vi "Design a Fixed-Point Interpolation Multirate Filter.vi"() -> ()   [LabVIEW 2023]
uses:
  <vilib>/addons/Digital Filter Design/FXPMRateSim.llb/DFD FXP MRate Simulation (DBL).vi
  <vilib>/addons/Digital Filter Design/FilterLib.llb/DFD Save MRate Filter to File.vi
  <vilib>/addons/Digital Filter Design/NI_DigFilterLicensed.lvlib
panel:
  out "Error Message":string
  in  "Save Filter to File":bool
  in  "Signal from DAQ Device":fxp<+/-,20,5>[](array[numeric])=[-0.329681396484375, -4.286834716796875, 9.429473876953125, -8.305145263671875, -0.662689208984375, -2.729522705078125, 7.085845947265625, -3.488800048828125, 2.225128173828125, 3.63323974609375, -5.179962158203125, 7.238677978515625, 4.8243408203125, 2.791412353515625, -9.072296142578125, -1.45458984375, 9.80548095703125, 7.69830322265625, -9.72210693359375, 1.994598388671875, -6.56597900390625, 5.69097900390625, 8.246246337890625, -2.866546630859375, -6.74896240234375, -7.206298828125, -4.030517578125, 6.043731689453125, 8.05010986328125, 3.516815185546875, 9.917205810546875, -8.699188232421875, 0.4688720703125, 0.513763427734375, 4.93695068359375, 5.129974365234375, -7.52783203125, 7.8001708984375, 1.576171875, 2.575714111328125, -4.20550537109375, -1.79620361328125, -5.672332763671875, 7.192901611328125, 9.375030517578125, -2.6258544921875, -5.70220947265625, 4.27691650390625, -0.683868408203125, 4.7548828125, 7.179962158203125, 7.098846435546875, -4.2564697265625, -8.908050537109375, -3.31884765625, 5.65350341796875, 0.428924560546875, 1.617706298828125, 7.4306640625, 4.920562744140625, -7.7008056640625, -7.17559814453125, -4.438934326171875, 8.03948974609375, 6.6856689453125, -2.220062255859375, -5.266357421875, -9.69549560546875, -7.25823974609375, 3.82177734375, 6.288909912109375, -1.042572021484375, 1.600128173828125, 8.114593505859375, 3.807037353515625, 7.95660400390625, -4.94366455078125, 0.53521728515625, 5.354522705078125, 5.111419677734375, 5.87420654296875, 5.844146728515625, 7.76446533203125, 6.58843994140625, 2.994964599609375, 0.97381591796875, 4.075286865234375, -2.38446044921875, -8.872802734375, 7.240264892578125, 3.440216064453125, -3.22064208984375, 7.457244873046875, -8.672027587890625, -7.299957275390625, -7.650421142578125, -8.7384033203125, -2.68670654296875, -0.992645263671875, 7.793701171875, -7.697601318359375, -1.930633544921875, 7.630767822265625, 8.330291748046875, -8.08685302734375, -8.128021240234375, 2.206024169921875, -2.2911376953125, -7.6170654296875, -6.148284912109375, -9.52166748046875, -5.676300048828125, 9.081939697265625, -1.682403564453125, -0.28973388671875, 2.24139404296875, -2.659698486328125, -9.855255126953125, 1.220489501953125, 2.930938720703125, 9.869171142578125, -2.096160888671875, 4.275848388671875, 0.7493896484375, 7.155364990234375, 8.169921875, 2.828765869140625, 8.2470703125] format="%.6g"
  out "Filtered Signals":dbl[](graph)
  # "Design a fixed-point highpass interpolation filter"
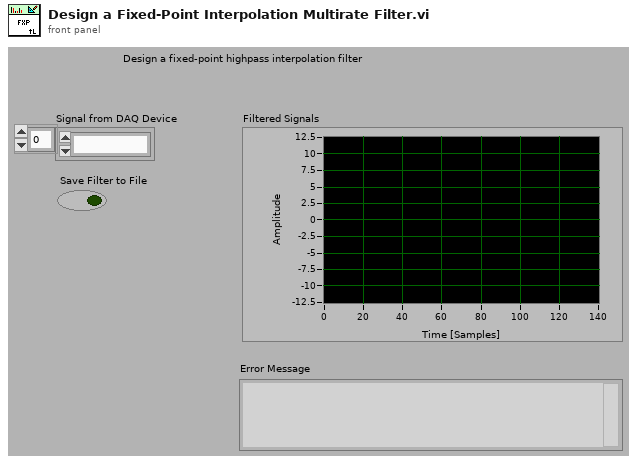
[diagram p1: front panel]
types:
  T1 = typedef "NI_DigFilterLicensed.lvlib/DFD Multirate Filter Obj.ctl" = cluster{"mMRate_Structure":enum16{"CIC", "FIR", "IIR", "Lattice"}, "mMRate_Mode":T2, "mMRate_Factor":i32, "mMRate_FIRParams":cluster{"mMRate_FIR_H":dbl[], "mMRate_FIR_IsNyquist?":bool, "mMRate_FIR_IsSymmetric?":bool}, "mMRate_CICParams":cluster{"mMRate_CIC_#Stage":i32, "mMRate_CIC_Lag":i32, "mMRate_CIC_Type":enum16{"Lowpass", "Highpass"}}, "mMRate_Order":i32, "mMRate_Version":string, "mMRate_Comments":string, "mMRate_RationalFactor":cluster{"mMRate_L":i32, "mMRate_M":i32}, "mMRate_Fs":dbl, "mMRate_Quantized?":bool, "mMRate_QFilterGain":dbl, "mMRate_CoefWl":i16, "mMRate_Scaling":cluster{"mMRate_ScaleByPowerOf2?":bool, "mMRate_ScaleType":T3}, "mMRate_InputWl":i16, "mMRate_OutputWl":i16, "mMRate_OutputMode":T4, "mMRate_MultMode":T5, "mMRate_BitPruning":bool, "mMRate_GainWl":i16, "mMRate_OutputFwl":i16, "mMRate_SumIwl":i16, "mMRate_InputIwl ":i16, "mMRate_SumWl":i16, "mMRate_CoefIwl":i16}
  T2 = typedef "NI_DigFilterLicensed.lvlib/DFD Multirate Mode.ctl" = i16
  T3 = typedef "NI_DigFilterLicensed.lvlib/DFD Coef Norm Type.ctl" = enum16{"No Norm", "Time Domain 1-Norm", "Time Domain 2-Norm", "Time Domain Inf-Norm"}
  T4 = typedef "NI_DigFilterLicensed.lvlib/DFD Round-off Mode.ctl" = enum16{"Nearest", "Truncation"}
  T5 = typedef "NI_DigFilterLicensed.lvlib/DFD FXP MRate Multiply Mode.ctl" = enum16{"Truncated", "Full"}
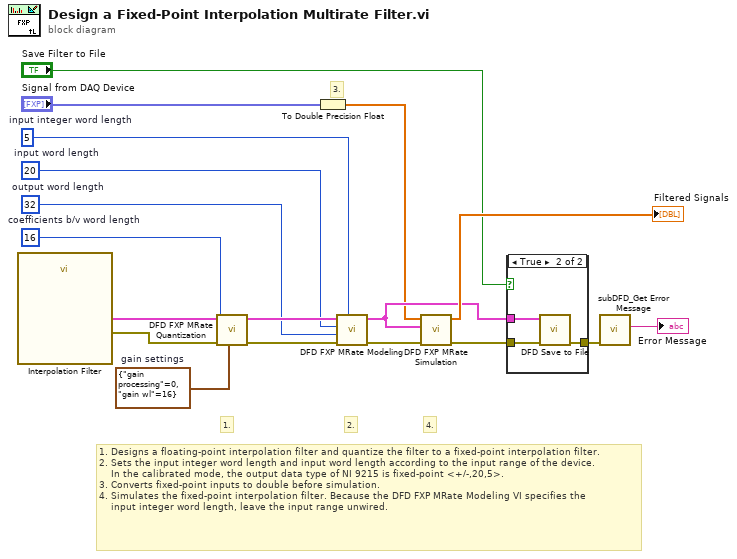
[diagram p0: block diagram]
diagram:
  w11 = i16 5  # input integer word length
  w12 = i16 32  # output word length
  w13 = i16 20  # input word length
  w16 = i16 16  # coefficients b/v word length
  w15 = cluster{"gain processing":u16, "gain wl":i16} {"gain processing"=0, "gain wl"=16}  # gain settings
  # "3."
  # "1."
  # "4."
  # "2."
  # "1. Designs a floating-point interpolation filter and quantize the filter to a fixed-point interpolation filter.\n2. Sets the input integer word length and input word length according to the input range of the device.\n    In the calibrated mode, the output data type of NI 9215 is fixed-point <+/-,20,5>.\n3. Converts fixed-point inputs to double before simulation. \n4. Simulates the fixed-point interpolation filter. Because the DFD FXP MRate Modeling VI specifies the \n    input integer word length, leave the input range unwired."
  n1 = call "Interpolation Filter"() -> ("error out"=w3:errorcluster, "multirate filter out"=w4:T1)  [unwired: 10 out]
  n2 = call <vilib>:"DFD FXP MRate Quantization.vi"("gain settings"=w15, "error in (no error)"=w3, "coefficients word length"=w16, "multirate filter in"=w4) -> ("error out"=w17:errorcluster, "multirate filter out"=w18:T1)  [unwired: 2 in, 4 out]
  n3 = To Double Precision Float(number="Signal from DAQ Device") -> (double precision float=w1:dbl[])
  n4 = call <vilib>:"DFD FXP MRate Modeling.vi"("input integer word length"=w11, "error in (no error)"=w17, "output word length"=w12, "input word length"=w13, "multirate filter in"=w18) -> ("error out"=w14:errorcluster, "multirate filter out"=w7:T1)  [unwired: 3 in, 2 out]
  n5 = call-poly <vilib>:"DFD FXP MRate Simulation.vi"("error in (no error)"=w14, "multirate filter"=w7, "signal in"=w1) -> ("error out"=w8:errorcluster, "DBL signal out"=→"Filtered Signals":dbl[])  [unwired: 2 in, 5 out]
  n6 = case shown="True" "Save Filter to File" {
    tunnel: w8 -> [w19 w22]
    tunnel: w7 -> [_ w21]
    tunnel: [w19 w20] -> w5
    frame False {
    }
    frame True {
      n7 = call-poly <vilib>:"DFD Save to File.vi"("error in (no error)"=w22, "multirate filter in"=w21) -> ("error out"=w20:errorcluster)  [unwired: 2 in, 7 out]
    }
  }
  n8 = call <vilib>:"subDFD_Get Error Message.vi"("error in (no error)"=w5) -> ("Error Message"=→"Error Message":string)  [unwired: 10 out]
